vi "Receive Message.vi"(6 "timeout in ms (-1)":i32=-1, 8 "error in":errorcluster, 11 "UserEventMessageTransport":refnum<class "UserEventMessageTransport.lvclass">) -> (0 "error out":errorcluster, 2 "User Event":refnum<class "IMessagePayload.lvclass">, 3 "UserEventMessageTransport out":refnum<class "UserEventMessageTransport.lvclass">)   [LabVIEW 2016, in "UserEventMessageTransport.lvclass"]
uses:
  UserEventMessageTransport.lvclass
  IMessagePayload/IMessagePayload.lvclass
  QMHMessagePayload/QMHMessagePayload.lvclass
  UserEventMessageTransport.lvclass/UserEventMessageTransport.ctl
panel:
  # "INPUTS"
  # "OUTPUTS"
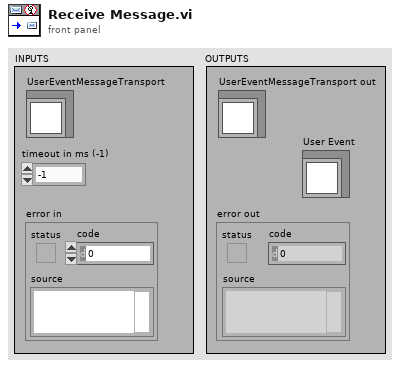
[diagram p1: front panel]
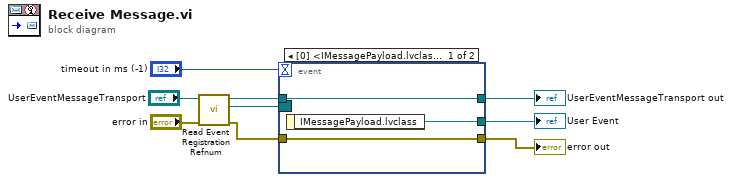
[diagram p0: block diagram]
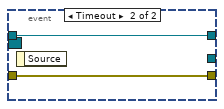
[diagram p2: hidden frame]
diagram:
  n1 = call "Read Event Registration Refnum.vi"("error in"="error in", "UserEventMessageTransport in"="UserEventMessageTransport") -> ("error out"=w4:errorcluster, "Event Registration Refnum"=w6:refnum<event-registration>, "UserEventMessageTransport out"=w2:refnum<class "UserEventMessageTransport.lvclass">)  [unwired: 7 in]
  n2 = event shown="[0] <IMessagePayload.lvclass>: User Event" {
    selector: w6 -> [_ _]
    dyn-events: _ -> [_ _]
    timeout: "timeout in ms (-1)" -> [_ _]
    tunnel: [w12 _] -> w5
    tunnel: w4 -> [w11 w13]
    tunnel: [w11 w13] -> w3
    tunnel: w2 -> [w10 w14]
    tunnel: [w10 w14] -> w1
    event User Event {
      n3 = event-data() -> ("IMessagePayload.lvclass"=w12:refnum<class "IMessagePayload.lvclass">)  [unwired: 1 in]
    }
    event Timeout {
      n4 = event-data() -> ()  [unwired: 1 in, 1 out]
    }
  }
  "error out" <- w3
  "UserEventMessageTransport out" <- w1
  "User Event" <- w5
